vi "get hdf device list.vi"(9 "nDevices":i32, 10 "monitor_ids":string, 11 "file":string) -> (1 "nDevices out":i32, 2 "monitor_ids out":string, 3 "file out":string, 5 "function return":i32)   [LabVIEW 2019, in "apdm.lvlib"]
doc: "APDM_EXPORT int apdm_get_hdf_device_list(char *file, char **monitor_ids, int *nDevices);"
uses:
  apdm.lvlib
  Lee Lab/CP FES Walking 2018/Code/Working/LabVIEW/apdm.dll
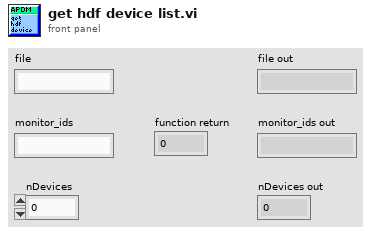
[diagram p1: front panel]
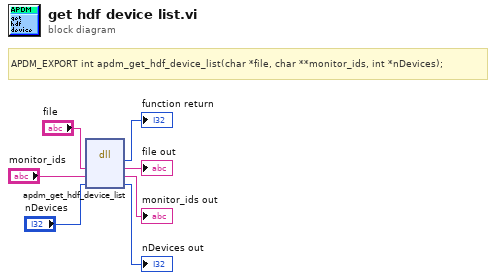
[diagram p0: block diagram]
diagram:
  # "APDM_EXPORT\tint apdm_get_hdf_device_list(char *file, char **monitor_ids, int *nDevices);"
  n1 = dll-call lib="C:/Users/jfalesi/Dropbox/Lee Lab/CP FES Walking 2018/Code/Working/LabVIEW/apdm.*" fn="apdm_get_hdf_device_list"("file"="file", "monitor_ids"="monitor_ids", "nDevices"="nDevices") -> (→"function return":i32, "file"=→"file out":string, "monitor_ids"=→"monitor_ids out":string, "nDevices"=→"nDevices out":i32)  [unwired: 3 in, 2 out]
